vi "Process Valve Mode Command (SubVI).vi"(4 "Valve Mode In":string, 6 "Address":string, 8 "error in (no error)":errorcluster, 11 "VISA Refnum in":refnum<visa-resource-name>) -> (0 "error out":errorcluster, 2 "Valve Mode Out":string, 3 "VISA Refnum out":refnum<visa-resource-name>)   [LabVIEW 2020]
doc: "Reads/writes instrument's valve operational mode. Leave \"Valve Mode In\" input terminal open to read current status. Wire to \"Valve Mode In\" input terminal following string:\nC - Close Valve\nA - Auto (normal operational mode to control setpoint). \nO - Open Valve\nWARNING: Before activating Valve Open mode make sure the differential pressure across instrument does not exceed maximum allowed differential pressure for corresponding DPM/DPC model (12 PSID for regular instruments and 9.75 PSID for low differential pressure BREEZE models)."
uses:
  <vilib>/Instr/_visa.llb/VISA Flush IO Buffer Mask.ctl
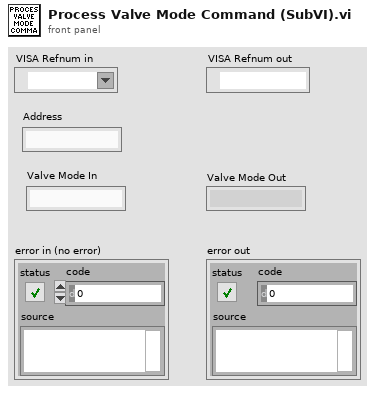
[diagram p1: front panel]
types:
  T1 = typedef "VISA Flush IO Buffer Mask.ctl" = u16
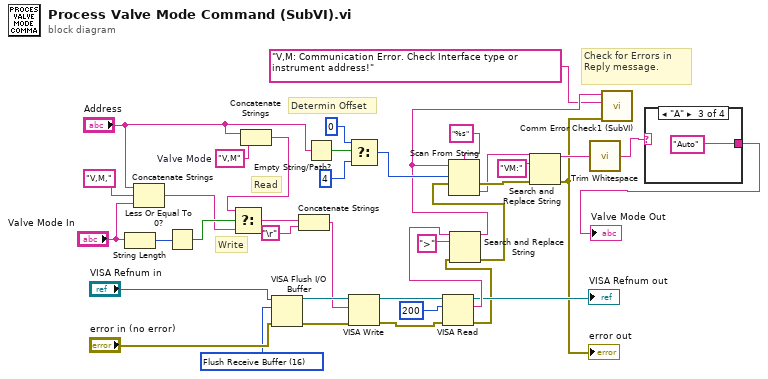
[diagram p0: block diagram]
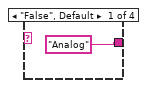
[diagram p2: hidden frame]
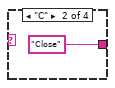
[diagram p3: hidden frame]
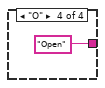
[diagram p4: hidden frame]
diagram:
  w26 = "V,M"  # Valve Mode
  w27 = T1 16 items=["Flush Receive Buffer"=16, "Write Transmit Buffer to Device"=32, "Flush Receive Buffer (No I/O)"=64, "Flush Transmit Buffer"=128] ("Mask")
  # "Write"
  # "Read"
  # "Check for Errors in Reply message."
  # "Determin Offset"
  n1 = String Length(string="Valve Mode In") -> (length=w10:i32)
  n2 = Concatenate Strings("Address", "V,M,", "Valve Mode In") -> (w6:string)
  n3 = Less Or Equal To 0?(x=w10) -> (x <= 0?=w9:bool)
  n4 = Concatenate Strings("Address", w26) -> (w14:string)
  n5 = Select(t=w14, s=w9, f=w6) -> (s? t:f=w13:string)
  n6 = VISA Flush I/O Buffer(VISA resource name="VISA Refnum in", mask (16)=w27, error in (no error)="error in (no error)") -> (VISA resource name out=w32:refnum<visa-resource-name>, error out=w12:errorcluster)
  n7 = Concatenate Strings(w13, "\r") -> (w31:string)
  n8 = Empty String/Path?(string/path="Address") -> (empty?=w23:bool)
  n9 = Select(t=0, s=w23, f=4) -> (s? t:f=w16:i32)
  n10 = VISA Write(VISA resource name=w32, write buffer=w31, error in (no error)=w12) -> (VISA resource name out=w34:refnum<visa-resource-name>, error out=w38:errorcluster)  [unwired: 1 out]
  n11 = VISA Read(VISA resource name=w34, byte count=200, error in (no error)=w38) -> (VISA resource name out=→"VISA Refnum out":refnum<visa-resource-name>, read buffer=w37:string, error out=w19:errorcluster)  [unwired: 1 out]
  n12 = Search and Replace String(input string=w37, search string=">", error in=w19) -> (result string=w3:string, error out=w18:errorcluster)  [unwired: 5 in, 2 out]
  n13 = Scan From String(format string="%s", input string=w3, initial scan location=w16, error in=w18) -> (error out=w17:errorcluster, output 1=w15:string)  [unwired: 1 in, 2 out]
  n14 = Search and Replace String(input string=w15, search string="VM:", error in=w17) -> (result string=w24:string, error out=w1:errorcluster)  [unwired: 5 in, 2 out]
  "error out" <- w1
  n15 = call <vilib>:"Trim Whitespace.vi"("string"=w24) -> ("trimmed string"=w5:string)  [unwired: 1 in]
  n16 = call "Comm Error Check1 (SubVI).vi"("error in (no error)"=w1, "Error Source String"="V,M: Communication Error. Check Interface type or instrument address!", "result string"=w3) -> ()  [unwired: 9 in]
  n17 = case shown="\"A\"" w5 {
    tunnel: ["Analog" "Close" "Auto" "Open"] -> w4
    frame "False", Default {
    }
    frame "C" {
    }
    frame "A" {
    }
    frame "O" {
    }
  }
  "Valve Mode Out" <- w4
